vi "rotateText.vi"(8 "error in (no error)":errorcluster, 9 "textIn":string, 11 "TextDisplay Class in":refnum<class "TextDisplay Class.lvclass">) -> (0 "error out":errorcluster, 3 "TextDisplay Class out":refnum<class "TextDisplay Class.lvclass">)   [LabVIEW 2019, in "TextDisplay Class.lvclass"]
uses:
  TextDisplay Class.lvclass
  TextDisplay Class.lvclass/TextDisplay Class.ctl
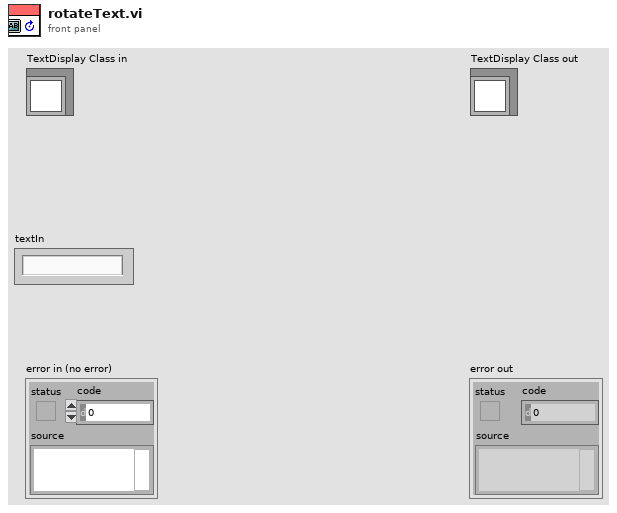
[diagram p1: front panel]
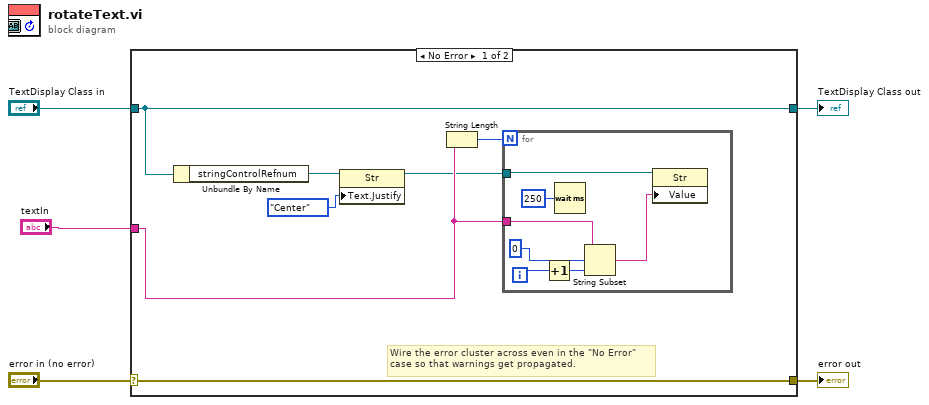
[diagram p0: block diagram]
diagram:
  n1 = case shown="No Error" "error in (no error)" {
    selector: "error in (no error)" -> [w12 w21]
    tunnel: [w12 w21] -> w4
    tunnel: [w10 w20] -> w2
    tunnel: "TextDisplay Class in" -> [w10 w20]
    tunnel: "textIn" -> [w11 _]
    frame No Error {
      # "Wire the error cluster across even in the \"No Error\"\ncase so that warnings get propagated."
      n2 = Unbundle By Name(w10) -> ("stringControlRefnum"=w9:refnum<vi>)
      n3 = property on="Property Node" class="Str"(reference=w9, "Text.Justify"=enum16{"Left", "Center", "Right"}."Center" ("Text.Justification")) -> (reference out=w7:refnum<vi>)  [unwired: 1 in, 1 out]
      n4 = String Length(string=w11) -> (length=w6:i32)
      n5 = for {
        N: w6 -> [_]
        tunnel: w11 -> [w16]
        tunnel: w7 -> [w14]
        i -> [w17]
        n6 = Increment(x=w17) -> (x+1=w15:i32)
        n7 = Wait (ms)(milliseconds to wait=u32 250) -> ()  [unwired: 1 out]
        n8 = String Subset(string=w16, offset (0)=0, length (rest)=w15) -> (substring=w13:string)
        n9 = property class="Str"(reference=w14, "Value"=w13) -> ()  [unwired: 1 in, 2 out]
      }
    }
    frame Error {
    }
  }
  "error out" <- w4
  "TextDisplay Class out" <- w2
